vi "InjB-FPGA.vi"() -> ()   [LabVIEW 2016]
uses:
  Glassman Readback.ctl
  Aperture Readback.ctl
  Glassman Control.ctl
  <vilib>/LabVIEW Targets/FPGA/cRIO/shared/nicrio_ModuleControls/nicrio_cRIO-9871_BaudRateEnum.ctl
  <vilib>/LabVIEW Targets/FPGA/cRIO/shared/nicrio_ModuleControls/nicrio_cRIO-9871_DataBitsEnum.ctl
  <vilib>/LabVIEW Targets/FPGA/cRIO/shared/nicrio_ModuleControls/nicrio_cRIO-9871_ParityEnum.ctl
  <vilib>/LabVIEW Targets/FPGA/cRIO/shared/nicrio_ModuleControls/nicrio_cRIO-9871_StopBitsEnum.ctl
  <vilib>/rvi/Emulation/niFpgaGetClockAttributes.vi
  <vilib>/rvi/Emulation/niFpgaSctlEmulationGetInTimedLoop.vi
  <vilib>/rvi/Emulation/niFpgaEmulationReportErrorSimple.vi
  <vilib>/rvi/eio/common/nirviEmuTemplateMethod_errors.vi
  <vilib>/rvi/Emulation/niFpgaCriticalErrorInLSC.vi
  <vilib>/rvi/eio/common/nirviEmuTemplatePropertySet_noerrors.vi
  <vilib>/eio/EIONode/EIONode.xnode
  <vilib>/eio/EIOMethodNode/EIOMethodNode.xnode
  <vilib>/eio/EIOPropertyNode/EIOPropertyNode.xnode
  <vilib>/rvi/eio/common/nirviEmuTemplatePropertyGet_errors.vi
  <vilib>/rvi/eio/common/nirviEmuTemplatePropertyGet_noerrors.vi
  <vilib>/rvi/eio/common/nirviEmuTemplatePropertySet_errors.vi
panel:
  in  "Bounce PS Set Value":u8[](array[numeric])
  out "Bounce PS readback":u8[](array[numeric])
  out "Bounce PS response":u8[](array[numeric])
  out "Bounce B-field":u8[](array[numeric])
  out "Cryo 1st stage temp":u8[](array[numeric])
  out "Cryo On-time":u8[](array[numeric])
  out "Cryo status":u8[](array[numeric])
  out "Beamline CG2":u8[](array[numeric])
  out "Beamline IG2":u8[](array[numeric])
  out "Beamline CG1":u8[](array[numeric])
  out "Beamline IG1":u8[](array[numeric])
  out "Ion Source CG2":u8[](array[numeric])
  out "Ion Source IG2":u8[](array[numeric])
  out "Ion Source CG1":u8[](array[numeric])
  out "Ion Source IG1":u8[](array[numeric])
  in  "2nd Einzel Control":T1
  in  "1st Einzel Control":T1
  in  "Extractor Control":T1
  out "2nd Einzel":T2
  out "Extractor":T2
  out "1st Einzel":T2
  out "V-monitor - X-steerer":fxp<+/-,26,5>
  out "I-monitor - X-steerer":fxp<+/-,26,5>
  out "V-monitor - Y-steerer":fxp<+/-,26,5>
  out "I-monitor - Y-steerer":fxp<+/-,26,5>
  in  "Voltage - Y-steerer":fxp<+/-,20,5>
  in  "Voltage - X-steerer":fxp<+/-,20,5>
  in  "Enable Y-steerer":bool
  in  "Enable X-steerer":bool
  out "I-monitor - TREK 10/40A":fxp<+/-,26,5>
  out "V-monitor - TREK 10/40A":fxp<+/-,26,5>
  out "Fault Status - TREK 10/40":bool
  out "Out-of-Regulation Status - TREK 10/40":bool
  in  "HV Enable - TREK 10/40":bool
  in  "Image Aperture Actuator":bool
  in  "BPM Aperture Actuator":bool
  in  "Object Aperture Actuator":bool
  out "BPM Aperture Sensors":T3
  out "Image Aperture Sensors":T3
  out "Object Aperture Sensors":T3
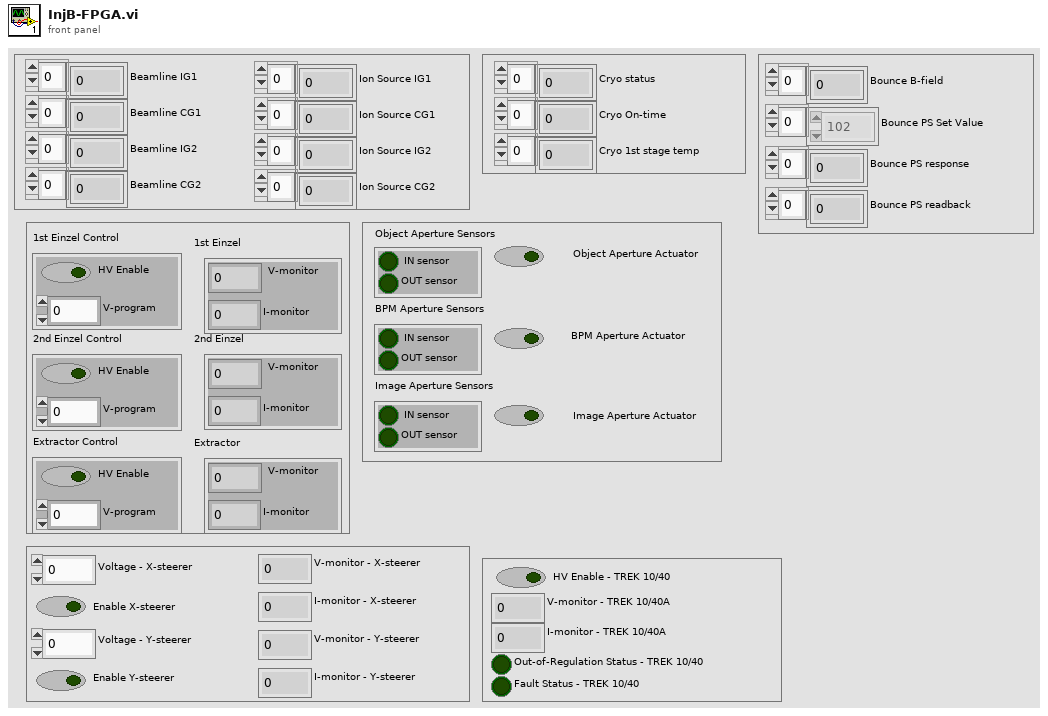
[diagram p1: front panel]
types:
  T1 = typedef "Glassman Control.ctl" = cluster{"V-program":fxp<+/-,20,5>, "HV Enable":bool}
  T2 = typedef "Glassman Readback.ctl" = cluster{"I-monitor":fxp<+/-,26,5>, "V-monitor":fxp<+/-,26,5>}
  T3 = typedef "Aperture Readback.ctl" = cluster{"IN sensor":bool, "OUT sensor":bool}
  T4 = typedef "nicrio_cRIO-9871_ParityEnum.ctl" = enum8{"None", "Odd", "Even", "Mark", "Space"}
  T5 = typedef "nicrio_cRIO-9871_StopBitsEnum.ctl" = enum8{"1", "1.5", "2"}
  T6 = typedef "nicrio_cRIO-9871_DataBitsEnum.ctl" = enum8{"5", "6", "7", "8"}
  T7 = typedef "nicrio_cRIO-9871_BaudRateEnum.ctl" = enum16{"75 bps", "110 bps", "134 bps", "150 bps", "300 bps", "600 bps", "1200 bps", "1800 bps", "2400 bps", "4800 bps", "7200 bps", "9600 bps", "14.4 kbps", "19.2 kbps", "28.8 kbps", "38.4 kbps", "57.6 kbps", "115.2 kbps", "230.4 kbps", "460.8 kbps", "921.6 kbps"}
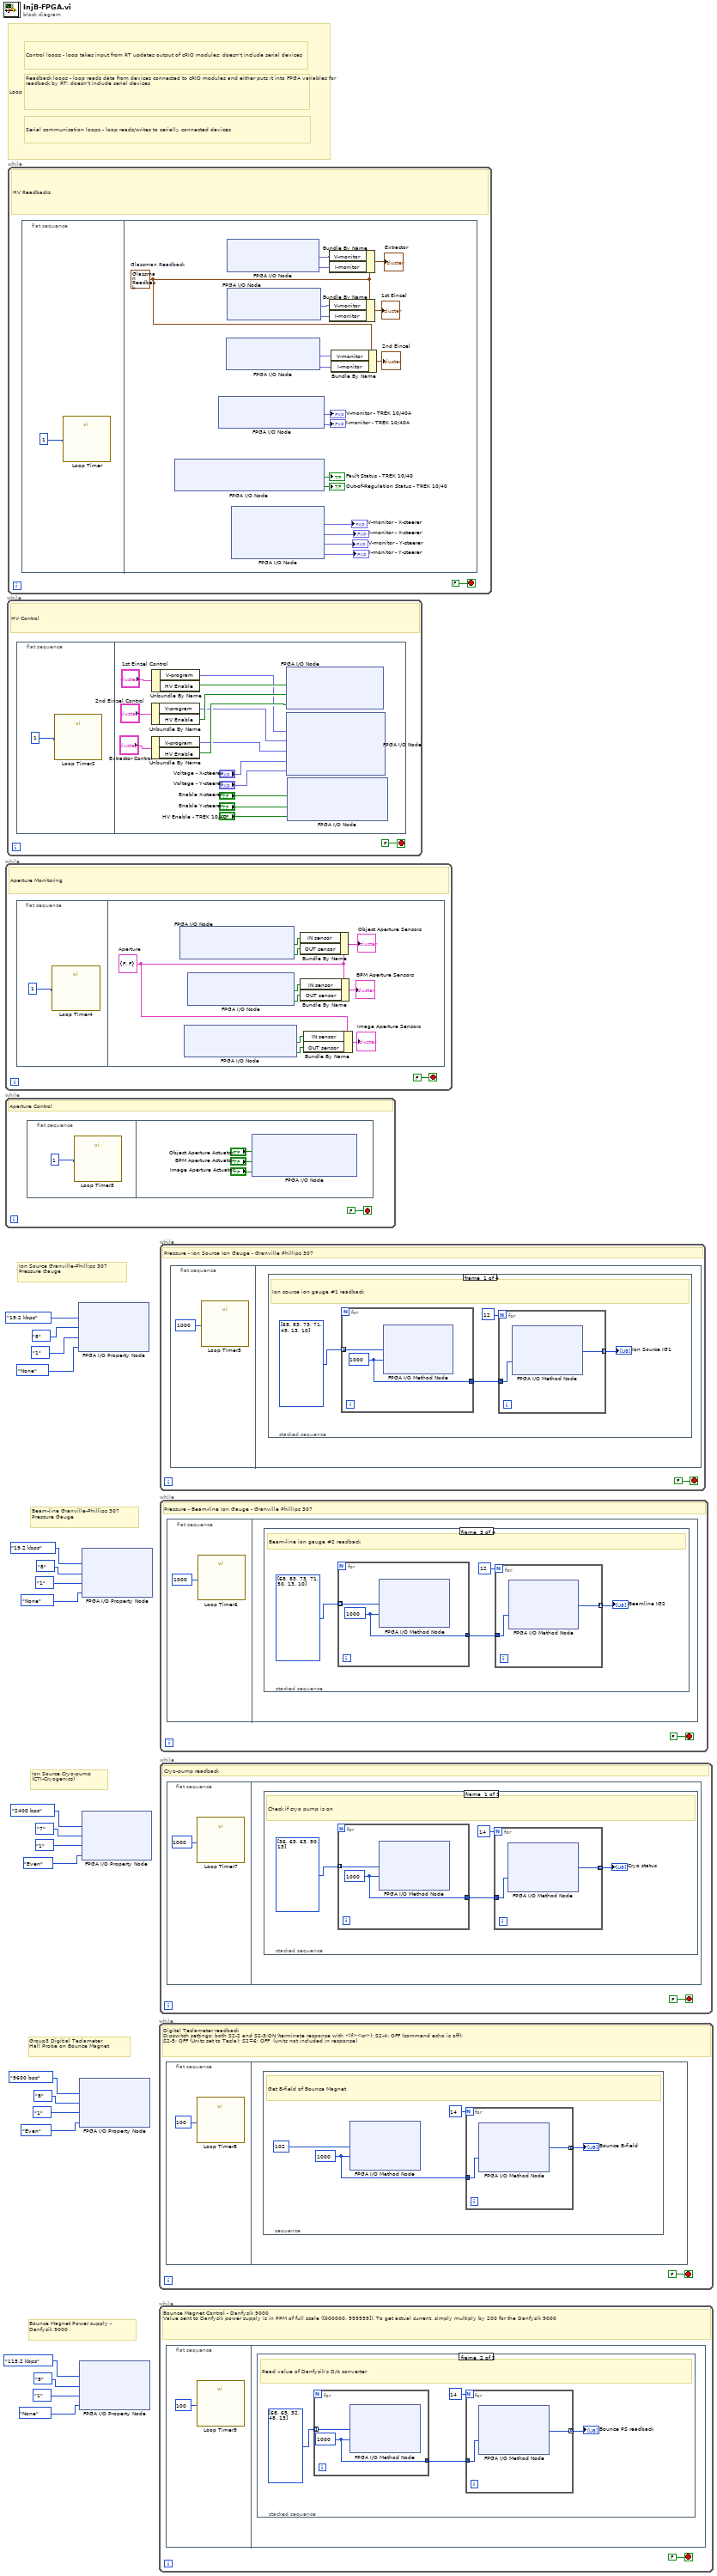
[diagram p0: block diagram]
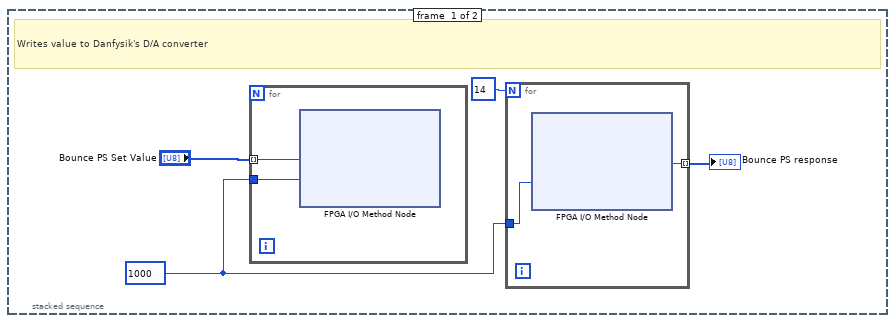
[diagram p2: hidden frame]
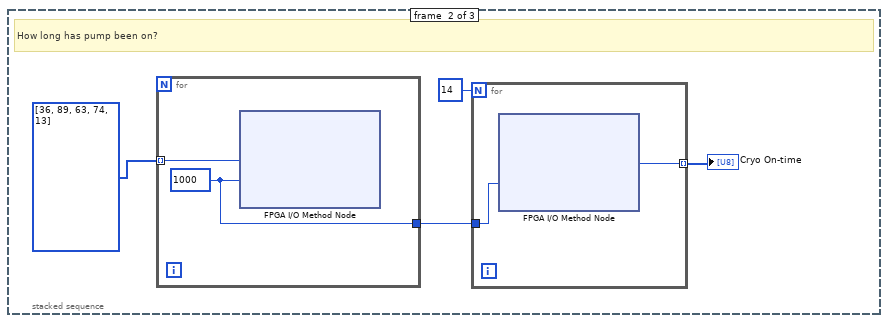
[diagram p3: hidden frame]
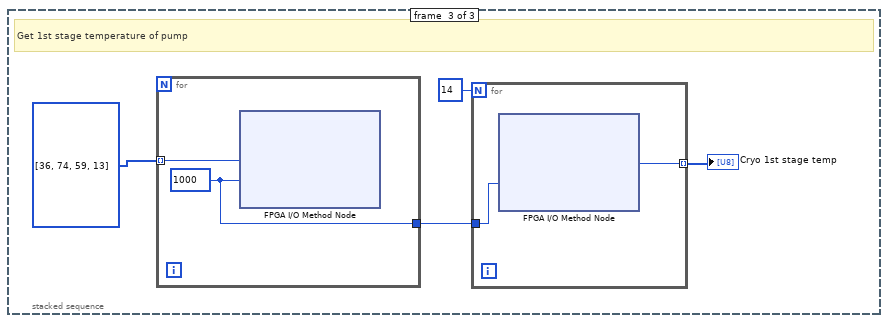
[diagram p4: hidden frame]
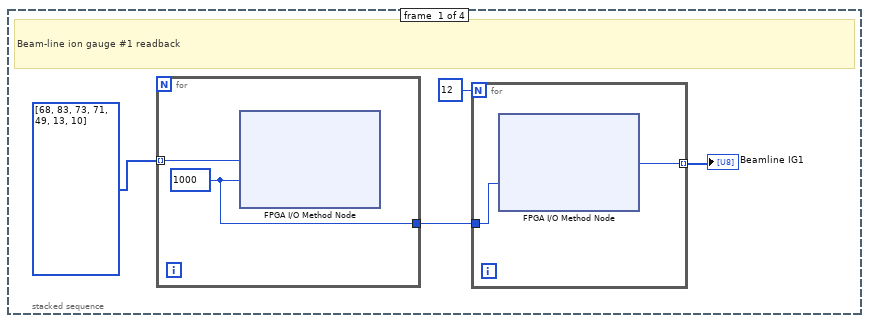
[diagram p5: hidden frame]
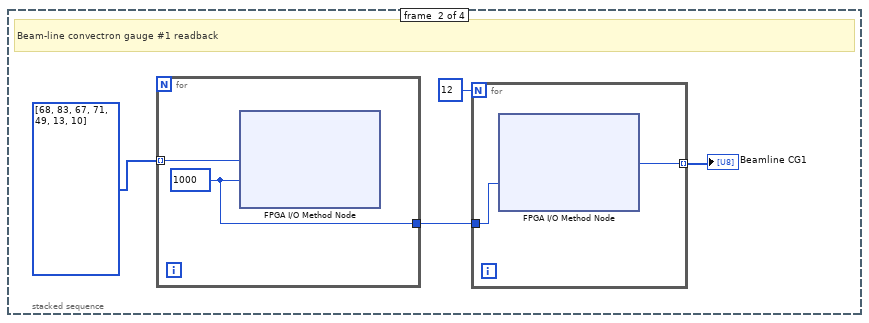
[diagram p6: hidden frame]
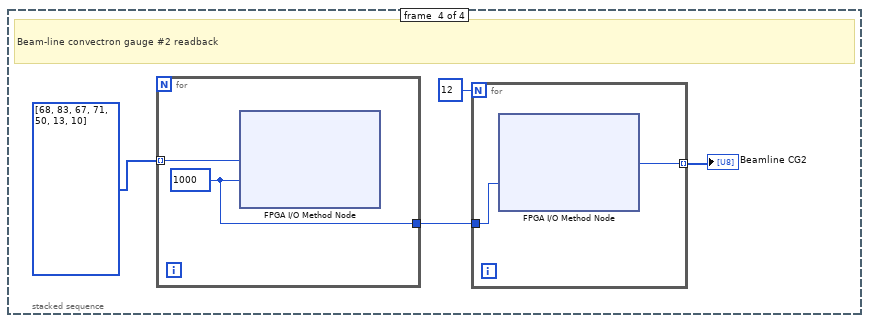
[diagram p7: hidden frame]
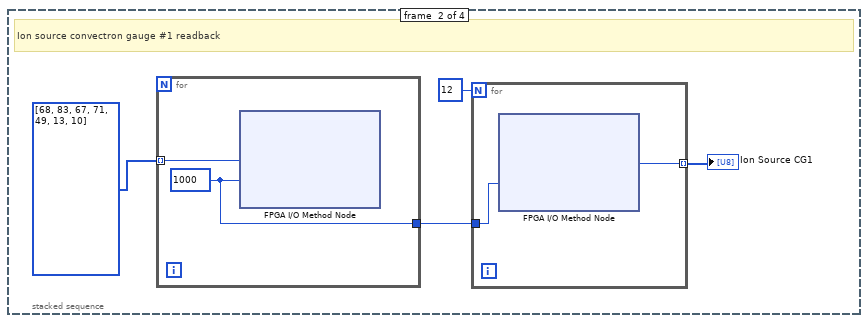
[diagram p8: hidden frame]
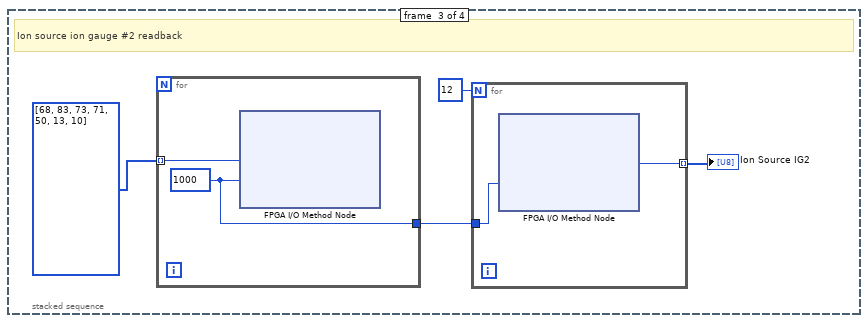
[diagram p9: hidden frame]
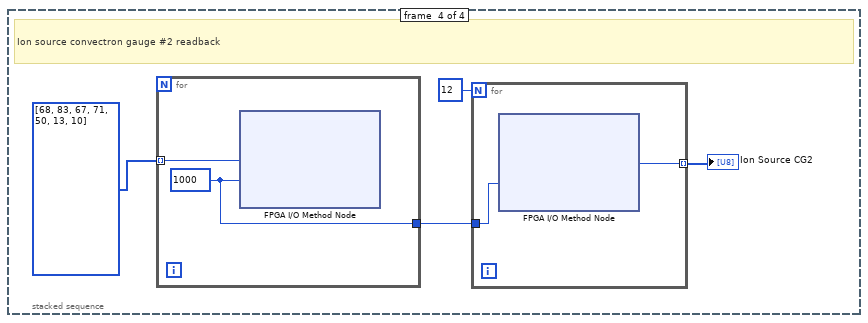
[diagram p10: hidden frame]
diagram:
  # "Bounce Magnet Power supply - \nDanfysik 9000"
  # "Group3 Digitial Teslameter\nHall Probe on Bounce Magnet"
  # "Ion Source Cryo-pump\n(CTI-Cryogenics)"
  # "Ion Source Granville-Phillips 307\nPressure Gauge"
  # "Beam-line Granville-Phillips 307\nPressure Gauge"
  # "Serial communication loops - loop reads/writes to serially connected devices"
  # "Readback loops - loop reads data from devices connected to cRIO modules and either puts it into FPGA variables for readback by RT; doesn't include serial devices"
  # "Control loops - loop takes input from RT updates output of cRIO modules; doesn't include serial devices"
  # "Loop legend - loops are color coded by responsibility"
  n1 = while {
    stop <- FALSE stop-if-true
    # "Aperture Control"
    n2 = flat-sequence {
      frame #0 {
        n3 = call "Loop Timer3"("Count(mSec)"=u32 1) -> ()  [unwired: 1 out]
      }
      frame #1 {
        n4 = xnode "FPGA I/O Node"("Object Aperture Actuator"="Object Aperture Actuator", "BPM Aperture Actuator"="BPM Aperture Actuator", "Image Aperture Actuator"="Image Aperture Actuator") -> ()  [unwired: 3 in, 3 out]
      }
    }
  }
  n5 = while {
    stop <- FALSE stop-if-true
    # "Aperture Monitoring"
    n6 = flat-sequence {
      frame #0 {
        n7 = call "Loop Timer4"("Count(mSec)"=u32 1) -> ()  [unwired: 1 out]
      }
      frame #1 {
        w28 = T3 {"IN sensor"=FALSE, "OUT sensor"=FALSE}  # Aperture
        n8 = xnode "FPGA I/O Node"() -> ("Object Aperture IN sensor"=w37:bool, "Object Aperture OUT sensor"=w36:bool)  [unwired: 2 in, 2 out]
        n9 = xnode "FPGA I/O Node"() -> ("Image Aperture IN sensor"=w33:bool, "Image Aperture OUT sensor"=w32:bool)  [unwired: 2 in, 2 out]
        n10 = xnode "FPGA I/O Node"() -> ("BPM Aperture IN sensor"=w35:bool, "BPM Aperture OUT sensor"=w34:bool)  [unwired: 2 in, 2 out]
        n11 = Bundle By Name(cluster=w28, "IN sensor"=w37, "OUT sensor"=w36) -> (→"Object Aperture Sensors":T3)
        n12 = Bundle By Name(cluster=w28, "IN sensor"=w35, "OUT sensor"=w34) -> (→"BPM Aperture Sensors":T3)
        n13 = Bundle By Name(cluster=w28, "IN sensor"=w33, "OUT sensor"=w32) -> (→"Image Aperture Sensors":T3)
      }
    }
  }
  n14 = while {
    stop <- FALSE stop-if-true
    # "HV Control"
    n15 = flat-sequence {
      frame #0 {
        n16 = call "Loop Timer2"("Count(mSec)"=u32 1) -> ()  [unwired: 1 out]
      }
      frame #1 {
        n17 = Unbundle By Name("2nd Einzel Control") -> ("V-program"=w41:fxp<+/-,20,5>, "HV Enable"=w44:bool)
        n18 = Unbundle By Name("Extractor Control") -> ("V-program"=w40:fxp<+/-,20,5>, "HV Enable"=w43:bool)
        n19 = Unbundle By Name("1st Einzel Control") -> ("V-program"=w42:fxp<+/-,20,5>, "HV Enable"=w45:bool)
        n20 = xnode "FPGA I/O Node"("HV Enable - 1st Einzel"=w45, "HV Enable - 2nd Einzel"=w44, "HV Enable - Extractor"=w43) -> ()  [unwired: 3 in, 3 out]
        n21 = xnode "FPGA I/O Node"("V-program - 1st Einzel"=w42, "V-program - 2nd Einzel"=w41, "V-program - Extractor"=w40, "Voltage - X-steerer"="Voltage - X-steerer", "Voltage - Y-steerer"="Voltage - Y-steerer") -> ()  [unwired: 5 in, 5 out]
        n22 = xnode "FPGA I/O Node"("Enable X-steerer"="Enable X-steerer", "Enable Y-steerer"="Enable Y-steerer", "HV Enable - TREK 10/40"="HV Enable - TREK 10/40") -> ()  [unwired: 3 in, 3 out]
      }
    }
  }
  n23 = while {
    stop <- FALSE stop-if-true
    # "HV Readbacks"
    n24 = flat-sequence {
      frame #0 {
        n25 = call "Loop Timer"("Count(mSec)"=u32 1) -> ()  [unwired: 1 out]
      }
      frame #1 {
        w60 = T2 {"I-monitor"=0.0, "V-monitor"=0.0}  # Glassman Readback
        n26 = xnode "FPGA I/O Node"() -> ("Fault Status - TREK 10/40"=→"Fault Status - TREK 10/40":bool, "Out-of-Regulation Status - TREK 10/40"=→"Out-of-Regulation Status - TREK 10/40":bool)  [unwired: 2 in, 2 out]
        n27 = xnode "FPGA I/O Node"() -> ("V-monitor - TREK 10/40A"=→"V-monitor - TREK 10/40A":fxp<+/-,26,5>, "I-monitor - TREK 10/40A"=→"I-monitor - TREK 10/40A":fxp<+/-,26,5>)  [unwired: 2 in, 2 out]
        n28 = xnode "FPGA I/O Node"() -> ("I-monitor - 1st Einzel"=w69:fxp<+/-,26,5>, "I-monitor - 2nd Einzel"=w68:fxp<+/-,26,5>)  [unwired: 2 in, 2 out]
        n29 = xnode "FPGA I/O Node"() -> ("V-monitor - Extractor"=w67:fxp<+/-,26,5>, "I-monitor - Extractor"=w66:fxp<+/-,26,5>)  [unwired: 2 in, 2 out]
        n30 = xnode "FPGA I/O Node"() -> ("V-monitor - 1st Einzel"=w65:fxp<+/-,26,5>, "I-monitor - 1st Einzel"=w64:fxp<+/-,26,5>)  [unwired: 2 in, 2 out]
        n31 = xnode "FPGA I/O Node"() -> ("V-monitor - X-steerer"=→"V-monitor - X-steerer":fxp<+/-,26,5>, "I-monitor - X-steerer"=→"I-monitor - X-steerer":fxp<+/-,26,5>, "V-monitor - Y-steerer"=→"V-monitor - Y-steerer":fxp<+/-,26,5>, "I-monitor - Y-steerer"=→"I-monitor - Y-steerer":fxp<+/-,26,5>)  [unwired: 4 in, 4 out]
        n32 = Bundle By Name(cluster=w60, "V-monitor"=w67, "I-monitor"=w66) -> (→"Extractor":T2)
        n33 = Bundle By Name(cluster=w60, "V-monitor"=w65, "I-monitor"=w64) -> (→"1st Einzel":T2)
        n34 = Bundle By Name(cluster=w60, "V-monitor"=w69, "I-monitor"=w68) -> (→"2nd Einzel":T2)
      }
    }
  }
  n35 = xnode "FPGA I/O Property Node"("Baud Rate"=nicrio_cRIO-9871_BaudRateEnum."19.2 kbps", "Data Bits"=nicrio_cRIO-9871_DataBitsEnum."8", "Stop Bits"=nicrio_cRIO-9871_StopBitsEnum."1", "Parity"=nicrio_cRIO-9871_ParityEnum."None") -> ()  [unwired: 1 in, 1 out]
  n36 = xnode "FPGA I/O Property Node"("Baud Rate"=nicrio_cRIO-9871_BaudRateEnum."9600 bps", "Data Bits"=nicrio_cRIO-9871_DataBitsEnum."8", "Stop Bits"=nicrio_cRIO-9871_StopBitsEnum."1", "Parity"=nicrio_cRIO-9871_ParityEnum."Even") -> ()  [unwired: 1 in, 1 out]
  n37 = xnode "FPGA I/O Property Node"("Baud Rate"=nicrio_cRIO-9871_BaudRateEnum."115.2 kbps", "Data Bits"=nicrio_cRIO-9871_DataBitsEnum."8", "Stop Bits"=nicrio_cRIO-9871_StopBitsEnum."1", "Parity"=nicrio_cRIO-9871_ParityEnum."None") -> ()  [unwired: 1 in, 1 out]
  n38 = xnode "FPGA I/O Property Node"("Baud Rate"=nicrio_cRIO-9871_BaudRateEnum."2400 bps", "Data Bits"=nicrio_cRIO-9871_DataBitsEnum."7", "Stop Bits"=nicrio_cRIO-9871_StopBitsEnum."1", "Parity"=nicrio_cRIO-9871_ParityEnum."Even") -> ()  [unwired: 1 in, 1 out]
  n39 = xnode "FPGA I/O Property Node"("Baud Rate"=nicrio_cRIO-9871_BaudRateEnum."19.2 kbps", "Data Bits"=nicrio_cRIO-9871_DataBitsEnum."8", "Stop Bits"=nicrio_cRIO-9871_StopBitsEnum."1", "Parity"=nicrio_cRIO-9871_ParityEnum."None") -> ()  [unwired: 1 in, 1 out]
  n40 = while {
    stop <- FALSE stop-if-true
    # "Digital Teslameter readback\nDipswitch settings: both S2-2 and S2-3:ON (terminate response with <lf><cr>); S2-4: OFF (command echo is off); \nS2-5: OFF (Units set to Tesla); S2=6: OFF  (units not included in response)"
    n41 = flat-sequence {
      frame #0 {
        n42 = call "Loop Timer8"("Count(mSec)"=u32 100) -> ()  [unwired: 1 out]
      }
      frame #1 {
        n43 = stacked-sequence {
          frame #0 {
            w78 = 1000 ("Timeout (ms)")
            # "Get B-field of Bounce Magnet"
            n44 = xnode "FPGA I/O Method Node"("Data"=u8 102, "Timeout (ms)"=w78) -> ()  [unwired: 1 in, 2 out]
            n45 = for {
              N: 14 -> [_]
              tunnel: [w81] -> w79 mode=indexing
              tunnel: w78 -> [w80]
              n46 = xnode "FPGA I/O Method Node"("Timeout (ms)"=w80) -> ("Data"=w81:u8)  [unwired: 1 in, 2 out]
            }
            "Bounce B-field" <- w79
          }
        }
      }
    }
  }
  n47 = while {
    stop <- FALSE stop-if-true
    # "Bounce Magnet Control - Danfysik 9000\nValue sent to Danfysik power supply is in PPM of full scale ([000000, 999999]). To get actual current, simply multiply by 200 for the Danfysik 9000"
    n48 = flat-sequence {
      frame #0 {
        n49 = call "Loop Timer9"("Count(mSec)"=u32 100) -> ()  [unwired: 1 out]
      }
      frame #1 {
        n50 = stacked-sequence {
          frame #0 {
            w85 = 1000 ("Timeout (ms)")
            # "Writes value to Danfysik's D/A converter"
            n51 = for {
              tunnel: w85 -> [w89]
              tunnel: "Bounce PS Set Value" -> [w88] mode=indexing
              n52 = xnode "FPGA I/O Method Node"("Data"=w88, "Timeout (ms)"=w89) -> ()  [unwired: 1 in, 2 out]
            }
            n53 = for {
              N: 14 -> [_]
              tunnel: [w91] -> w87 mode=indexing
              tunnel: w85 -> [w90]
              n54 = xnode "FPGA I/O Method Node"("Timeout (ms)"=w90) -> ("Data"=w91:u8)  [unwired: 1 in, 2 out]
            }
            "Bounce PS response" <- w87
          }
          frame #1 {
            # "Read value of Danfysik's D/A converter"
            n55 = for {
              tunnel: [w97] -> w94
              tunnel: u8[] [68, 65, 32, 48, 13] -> [w96] mode=indexing
              w97 = 1000 ("Timeout (ms)")
              n56 = xnode "FPGA I/O Method Node"("Data"=w96, "Timeout (ms)"=w97) -> ()  [unwired: 1 in, 2 out]
            }
            n57 = for {
              N: 14 -> [_]
              tunnel: [w99] -> w95 mode=indexing
              tunnel: w94 -> [w98]
              n58 = xnode "FPGA I/O Method Node"("Timeout (ms)"=w98) -> ("Data"=w99:u8)  [unwired: 1 in, 2 out]
            }
            "Bounce PS readback" <- w95
          }
        }
      }
    }
  }
  n59 = while {
    stop <- FALSE stop-if-true
    # "Pressure - Ion Source Ion Gauge - Granville Phillips 307"
    n60 = flat-sequence {
      frame #0 {
        n61 = call "Loop Timer5"("Count(mSec)"=u32 1000) -> ()  [unwired: 1 out]
      }
      frame #1 {
        n62 = stacked-sequence {
          frame #0 {
            # "Ion source ion gauge #1 readback"
            n63 = for {
              tunnel: u8[] [68, 83, 73, 71, 49, 13, 10] ("unsigned byte array") -> [w109] mode=indexing
              tunnel: [w108] -> w103
              w108 = 1000 ("Timeout (ms)")
              n64 = xnode "FPGA I/O Method Node"("Data"=w109, "Timeout (ms)"=w108) -> ()  [unwired: 1 in, 2 out]
            }
            n65 = for {
              N: 12 -> [_]
              tunnel: [w107] -> w105 mode=indexing
              tunnel: w103 -> [w106]
              n66 = xnode "FPGA I/O Method Node"("Timeout (ms)"=w106) -> ("Data"=w107:u8)  [unwired: 1 in, 2 out]
            }
            "Ion Source IG1" <- w105
          }
          frame #1 {
            # "Ion source convectron gauge #1 readback"
            n67 = for {
              tunnel: u8[] [68, 83, 67, 71, 49, 13, 10] ("unsigned byte array") -> [w117] mode=indexing
              tunnel: [w116] -> w111
              w116 = 1000 ("Timeout (ms)")
              n68 = xnode "FPGA I/O Method Node"("Data"=w117, "Timeout (ms)"=w116) -> ()  [unwired: 1 in, 2 out]
            }
            n69 = for {
              N: 12 -> [_]
              tunnel: [w115] -> w113 mode=indexing
              tunnel: w111 -> [w114]
              n70 = xnode "FPGA I/O Method Node"("Timeout (ms)"=w114) -> ("Data"=w115:u8)  [unwired: 1 in, 2 out]
            }
            "Ion Source CG1" <- w113
          }
          frame #2 {
            # "Ion source ion gauge #2 readback"
            n71 = for {
              tunnel: u8[] [68, 83, 73, 71, 50, 13, 10] ("unsigned byte array") -> [w125] mode=indexing
              tunnel: [w124] -> w119
              w124 = 1000 ("Timeout (ms)")
              n72 = xnode "FPGA I/O Method Node"("Data"=w125, "Timeout (ms)"=w124) -> ()  [unwired: 1 in, 2 out]
            }
            n73 = for {
              N: 12 -> [_]
              tunnel: [w123] -> w121 mode=indexing
              tunnel: w119 -> [w122]
              n74 = xnode "FPGA I/O Method Node"("Timeout (ms)"=w122) -> ("Data"=w123:u8)  [unwired: 1 in, 2 out]
            }
            "Ion Source IG2" <- w121
          }
          frame #3 {
            # "Ion source convectron gauge #2 readback"
            n75 = for {
              tunnel: u8[] [68, 83, 67, 71, 50, 13, 10] ("unsigned byte array") -> [w133] mode=indexing
              tunnel: [w132] -> w127
              w132 = 1000 ("Timeout (ms)")
              n76 = xnode "FPGA I/O Method Node"("Data"=w133, "Timeout (ms)"=w132) -> ()  [unwired: 1 in, 2 out]
            }
            n77 = for {
              N: 12 -> [_]
              tunnel: [w131] -> w129 mode=indexing
              tunnel: w127 -> [w130]
              n78 = xnode "FPGA I/O Method Node"("Timeout (ms)"=w130) -> ("Data"=w131:u8)  [unwired: 1 in, 2 out]
            }
            "Ion Source CG2" <- w129
          }
        }
      }
    }
  }
  n79 = while {
    stop <- FALSE stop-if-true
    # "Cryo-pump readback"
    n80 = flat-sequence {
      frame #0 {
        n81 = call "Loop Timer7"("Count(mSec)"=u32 1000) -> ()  [unwired: 1 out]
      }
      frame #1 {
        n82 = stacked-sequence {
          frame #0 {
            # "Check if cryo pump is on"
            n83 = for {
              tunnel: u8[] [36, 65, 63, 50, 13] ("unsigned byte array") -> [w143] mode=indexing
              tunnel: [w142] -> w137
              w142 = 1000 ("Timeout (ms)")
              n84 = xnode "FPGA I/O Method Node"("Data"=w143, "Timeout (ms)"=w142) -> ()  [unwired: 1 in, 2 out]
            }
            n85 = for {
              N: 14 -> [_]
              tunnel: [w141] -> w139 mode=indexing
              tunnel: w137 -> [w140]
              n86 = xnode "FPGA I/O Method Node"("Timeout (ms)"=w140) -> ("Data"=w141:u8)  [unwired: 1 in, 2 out]
            }
            "Cryo status" <- w139
          }
          frame #1 {
            # "How long has pump been on?"
            n87 = for {
              tunnel: u8[] [36, 89, 63, 74, 13] ("unsigned byte array") -> [w151] mode=indexing
              tunnel: [w150] -> w145
              w150 = 1000 ("Timeout (ms)")
              n88 = xnode "FPGA I/O Method Node"("Data"=w151, "Timeout (ms)"=w150) -> ()  [unwired: 1 in, 2 out]
            }
            n89 = for {
              N: 14 -> [_]
              tunnel: [w149] -> w147 mode=indexing
              tunnel: w145 -> [w148]
              n90 = xnode "FPGA I/O Method Node"("Timeout (ms)"=w148) -> ("Data"=w149:u8)  [unwired: 1 in, 2 out]
            }
            "Cryo On-time" <- w147
          }
          frame #2 {
            # "Get 1st stage temperature of pump"
            n91 = for {
              tunnel: u8[] [36, 74, 59, 13] ("unsigned byte array") -> [w159] mode=indexing
              tunnel: [w158] -> w153
              w158 = 1000 ("Timeout (ms)")
              n92 = xnode "FPGA I/O Method Node"("Data"=w159, "Timeout (ms)"=w158) -> ()  [unwired: 1 in, 2 out]
            }
            n93 = for {
              N: 14 -> [_]
              tunnel: [w157] -> w155 mode=indexing
              tunnel: w153 -> [w156]
              n94 = xnode "FPGA I/O Method Node"("Timeout (ms)"=w156) -> ("Data"=w157:u8)  [unwired: 1 in, 2 out]
            }
            "Cryo 1st stage temp" <- w155
          }
        }
      }
    }
  }
  n95 = while {
    stop <- FALSE stop-if-true
    # "Pressure - Beam-line Ion Gauge - Granville Phillips 307"
    n96 = flat-sequence {
      frame #0 {
        n97 = call "Loop Timer6"("Count(mSec)"=u32 1000) -> ()  [unwired: 1 out]
      }
      frame #1 {
        n98 = stacked-sequence {
          frame #0 {
            # "Beam-line ion gauge #1 readback"
            n99 = for {
              tunnel: u8[] [68, 83, 73, 71, 49, 13, 10] ("unsigned byte array") -> [w169] mode=indexing
              tunnel: [w168] -> w163
              w168 = 1000 ("Timeout (ms)")
              n100 = xnode "FPGA I/O Method Node"("Data"=w169, "Timeout (ms)"=w168) -> ()  [unwired: 1 in, 2 out]
            }
            n101 = for {
              N: 12 -> [_]
              tunnel: [w167] -> w165 mode=indexing
              tunnel: w163 -> [w166]
              n102 = xnode "FPGA I/O Method Node"("Timeout (ms)"=w166) -> ("Data"=w167:u8)  [unwired: 1 in, 2 out]
            }
            "Beamline IG1" <- w165
          }
          frame #1 {
            # "Beam-line convectron gauge #1 readback"
            n103 = for {
              tunnel: u8[] [68, 83, 67, 71, 49, 13, 10] ("unsigned byte array") -> [w177] mode=indexing
              tunnel: [w176] -> w171
              w176 = 1000 ("Timeout (ms)")
              n104 = xnode "FPGA I/O Method Node"("Data"=w177, "Timeout (ms)"=w176) -> ()  [unwired: 1 in, 2 out]
            }
            n105 = for {
              N: 12 -> [_]
              tunnel: [w175] -> w173 mode=indexing
              tunnel: w171 -> [w174]
              n106 = xnode "FPGA I/O Method Node"("Timeout (ms)"=w174) -> ("Data"=w175:u8)  [unwired: 1 in, 2 out]
            }
            "Beamline CG1" <- w173
          }
          frame #2 {
            # "Beam-line ion gauge #2 readback"
            n107 = for {
              tunnel: u8[] [68, 83, 73, 71, 50, 13, 10] ("unsigned byte array") -> [w185] mode=indexing
              tunnel: [w184] -> w179
              w184 = 1000 ("Timeout (ms)")
              n108 = xnode "FPGA I/O Method Node"("Data"=w185, "Timeout (ms)"=w184) -> ()  [unwired: 1 in, 2 out]
            }
            n109 = for {
              N: 12 -> [_]
              tunnel: [w183] -> w181 mode=indexing
              tunnel: w179 -> [w182]
              n110 = xnode "FPGA I/O Method Node"("Timeout (ms)"=w182) -> ("Data"=w183:u8)  [unwired: 1 in, 2 out]
            }
            "Beamline IG2" <- w181
          }
          frame #3 {
            # "Beam-line convectron gauge #2 readback"
            n111 = for {
              tunnel: u8[] [68, 83, 67, 71, 50, 13, 10] ("unsigned byte array") -> [w193] mode=indexing
              tunnel: [w192] -> w187
              w192 = 1000 ("Timeout (ms)")
              n112 = xnode "FPGA I/O Method Node"("Data"=w193, "Timeout (ms)"=w192) -> ()  [unwired: 1 in, 2 out]
            }
            n113 = for {
              N: 12 -> [_]
              tunnel: [w191] -> w189 mode=indexing
              tunnel: w187 -> [w190]
              n114 = xnode "FPGA I/O Method Node"("Timeout (ms)"=w190) -> ("Data"=w191:u8)  [unwired: 1 in, 2 out]
            }
            "Beamline CG2" <- w189
          }
        }
      }
    }
  }
